vi "Write Igus CanOpen.vi"(6 "Sub Index":u8 format="%.0x", 7 "Data [1-4]":u8[](array[numeric]) format="%.0x", 8 "error in (no error)":errorcluster, 10 "Address":u16 format="%.0x", 11 "MB session in":refnum<class "MB_Master.lvclass">) -> (0 "error out":errorcluster, 1 "Command":T1={"Function Code"=1, "Data"=[], "RTU_DataBytes"=0} {"Data" format="%.0x"}, 2 "Response":T1={"Function Code"=1, "Data"=[], "RTU_DataBytes"=0} {"Data" format="%.0x"}, 3 "MB session out":refnum<class "MB_Master.lvclass">)   [LabVIEW 2016, in "MB Master.lvlib"]
doc: "Function Code 43 / 14: Read device ID objects. Specify the type of access using the <b>read device ID code</b> and the id of the starting object using <b>object ID</b>.\n\nread device ID codes:\n 0x01 - Basic: Request the basic stream of devID objects (0x00 to 0x02) starting from the specified object ID.\n 0x02 - Regular: Requests the regular stream of devID objects (0x00 to 0x7F) starting from the specified object ID.\n 0x03 - Extended: Requests the extended stream of devID objects (0x00 to 0xFF) starting from the specified object ID.\n 0x04 - Single: Requests a single devID object specified by object ID.\n\nResponse is an array of devID objects. Each element contains the object ID and string value. The conformity level indicates the type of access supported by the device.\n\nConformity level values:\n0x01 - Basic (stream only)\n0x02 - Regular (stream only)\n0x03 - Extended (stream only)\n0x81 - Basic (stream and single)\n0x82 - Regular (stream and single)\n0x83 - Extended (stream and single)"
uses:
  MB Master.lvlib
  MB_Master.lvclass
  MB_PDU/MB_PDU_Cluster.ctl
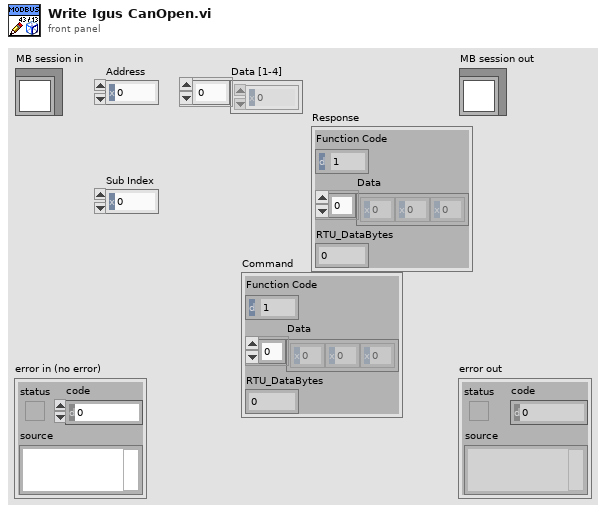
[diagram p1: front panel]
types:
  T1 = typedef "MB Master.lvlib/MB_PDU_Cluster.ctl" = cluster{"Function Code":u8, "Data":u8[], "RTU_DataBytes":i32}
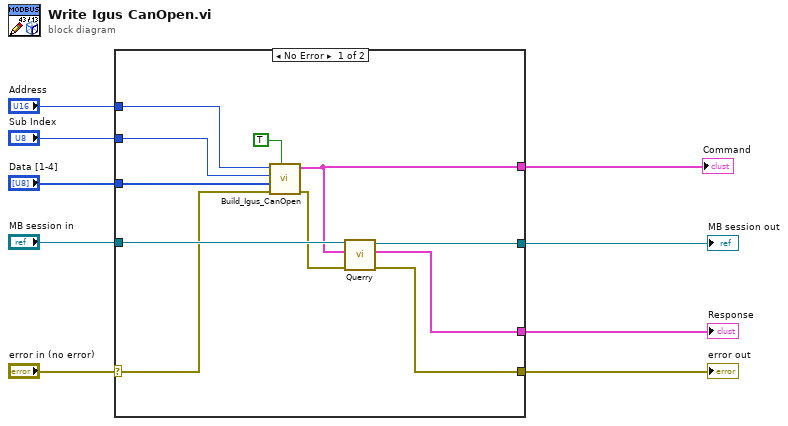
[diagram p0: block diagram]
diagram:
  n1 = case shown="No Error" "error in (no error)" {
    selector: "error in (no error)" -> [w18 w22]
    tunnel: [w17 w22] -> w8
    tunnel: [w20 w21] -> w6
    tunnel: "MB session in" -> [w19 w21]
    tunnel: [w16 _] -> w5
    tunnel: [w15 _] -> w4
    tunnel: "Address" -> [w12 _]
    tunnel: "Sub Index" -> [w11 _]
    tunnel: "Data [1-4]" -> [w10 _]
    frame No Error {
      n2 = call "Build_Igus_CanOpen.vi"("Read (F) / Write"=TRUE, "error in (no error)"=w18, "Data [1-4]"=w10, "Sub Index"=w11, "Address"=w12) -> ("error out"=w14:errorcluster, "MB_PDU"=w15:T1)  [unwired: 5 in]
      n3 = call-dynamic "Querry.vi"("error in (no error)"=w14, "PDU_req"=w15, "MB_Master in"=w19) -> ("error out"=w17:errorcluster, "PDU_resp"=w16:T1, "MB_Master out"=w20:refnum<class "MB_Master.lvclass">)  [unwired: 6 in]
    }
    frame Error {
    }
  }
  "error out" <- w8
  "MB session out" <- w6
  "Response" <- w5
  "Command" <- w4
